vi "从文件读命令.vi"(2 "Path":path, 3 "VISA error in":errorcluster, 4 "VISA resource name":refnum<visa-resource-name>) -> (0 "VISA error out":errorcluster, 1 "VISA resource name out":refnum<visa-resource-name>)   [LabVIEW 2018]
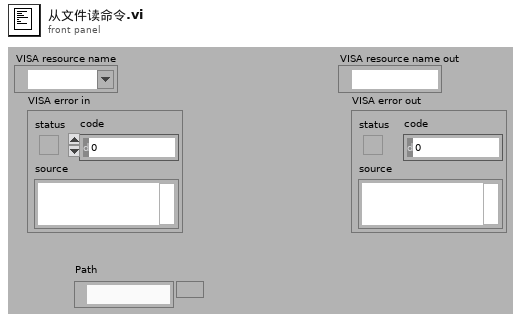
[diagram p1: front panel]
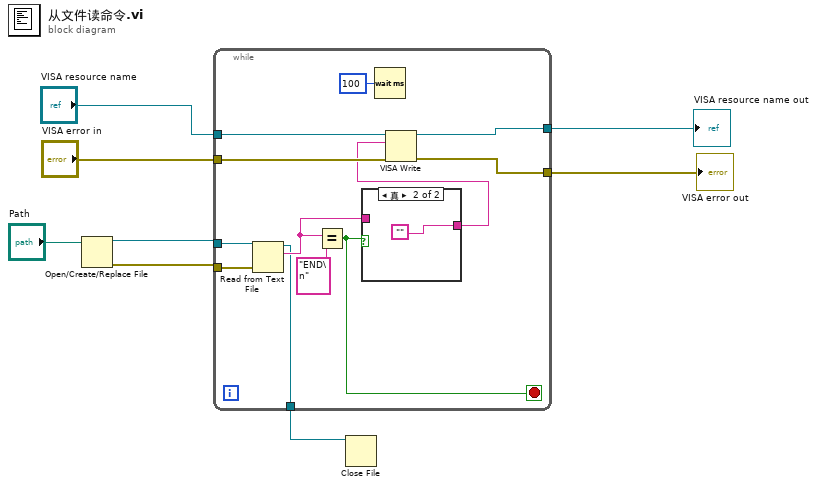
[diagram p0: block diagram]
diagram:
  n1 = Open/Create/Replace File(file path (use dialog)="Path") -> (refnum out=w6:refnum<file>, error out=w5:errorcluster)  [unwired: 5 in, 1 out]
  n2 = while {
    tunnel: "VISA resource name" -> [w20]
    tunnel: "VISA error in" -> [w19]
    tunnel: w6 -> [w18]
    tunnel: w5 -> [w17]
    tunnel: [w13] -> w4
    tunnel: [w12] -> w3
    tunnel: [w10] -> w2
    stop <- w11 stop-if-true
    n3 = Read from Text File(file (use dialog)=w18, error in=w17) -> (refnum out=w10:refnum<file>, text=w15:string)  [unwired: 2 in, 2 out]
    n4 = Equal?(x=w15, y="END\n") -> (x = y?=w11:bool)
    n5 = case shown="真" w11 {
      tunnel: w15 -> [w21 _]
      tunnel: [w21 ""] -> w14
      frame False {
      }
      frame True {
      }
    }
    n6 = Wait (ms)(milliseconds to wait=u32 100 ("等待时间（毫秒）")) -> ()  [unwired: 1 out]
    n7 = VISA Write(VISA resource name=w20, write buffer=w14, error in (no error)=w19) -> (VISA resource name out=w13:refnum<visa-resource-name>, error out=w12:errorcluster)  [unwired: 1 out]
  }
  "VISA resource name out" <- w4
  "VISA error out" <- w3
  n8 = Close File(refnum=w2) -> ()  [unwired: 1 in, 2 out]
